vi "FFT Filt.vi"(0 "Filter in":refnum<class "Filter.lvclass">, 5 "Y":dbl[](array[numeric]), 9 "Fs (Hz)":dbl, 11 "error in (no error)":errorcluster) -> (4 "Filter out":refnum<class "Filter.lvclass">, 6 "Yfilt":dbl[](array[numeric]), 10 "Gain":dbl, 15 "error out":errorcluster)   [LabVIEW 2020, in "Filter.lvclass"]
uses:
  Filter.lvclass
  Filter.lvclass/Filter.ctl
  Utility VIs/Math VIs/FFT x(t) to dB,Degrees (1D).vi
  Utility VIs/Math VIs/Z to dB, degrees (1D).vi
  Utility VIs/Math VIs/Linear to dB (scalar).vi
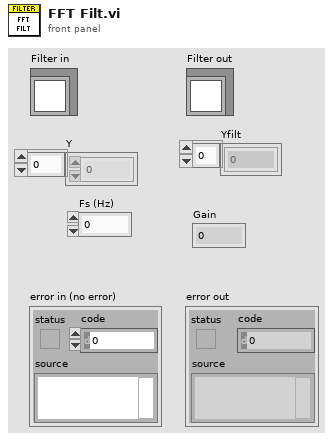
[diagram p1: front panel]
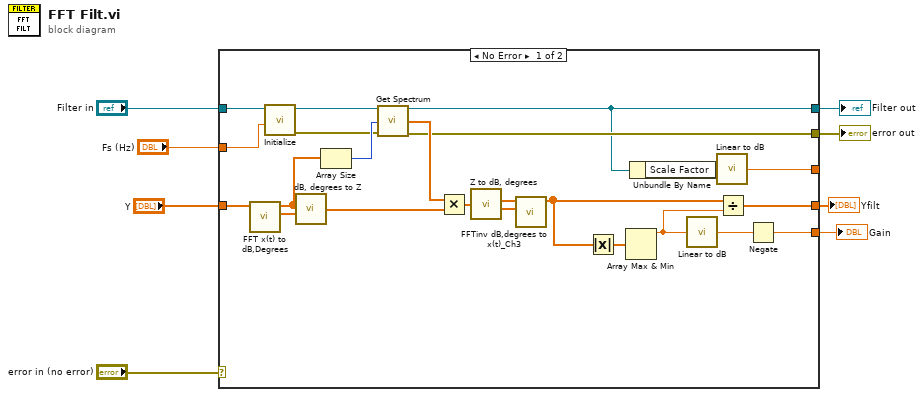
[diagram p0: block diagram]
diagram:
  n1 = case shown="No Error" "error in (no error)" {
    selector: "error in (no error)" -> [_ w33]
    tunnel: [w19 w33] -> w7
    tunnel: [w17 w32] -> w5
    tunnel: "Filter in" -> [w31 w32]
    tunnel: "Fs (Hz)" -> [w30 _]
    tunnel: "Y" -> [w28 _]
    tunnel: [w13 _] -> w2
    tunnel: [w12 _] -> _
    tunnel: [w9 _] -> w1
    frame No Error {
      n2 = call-poly "FFT x(t) to dB,Degrees.vi"("X"=w28) -> ("+Freq Phase of FFT (degrees)"=w26:dbl[], "+Freq. Mag of FFT (dB rms)"=w18:dbl[])  [unwired: 8 in, 1 out]
      n3 = call "Initialize.vi"("Fs (Hz)"=w30, "Filter in"=w31) -> ("error out"=w20:errorcluster, "Filter out"=w29:refnum<class "Filter.lvclass">)  [unwired: 8 in]
      n4 = call "dB, degrees to Z.vi"("Magnitude (dB)"=w18, "Phase (degrees)"=w26) -> ("Z"=w25:cdb[])  [unwired: 5 in]
      n5 = Array Size(array=w18) -> (size(s)=w27:i32)
      n6 = call "Get Spectrum.vi"("Filter in"=w29, "Npts"=w27, "error in (no error)"=w20) -> ("Filter out"=w17:refnum<class "Filter.lvclass">, "spectrum"=w24:cdb[], "error out"=w19:errorcluster)  [unwired: 10 in]
      n7 = Multiply(x=w24, y=w25) -> (x*y=w23:cdb[])
      n8 = call-poly "Z to dB, degrees.vi"("Z"=w23) -> ("Magnitude (dB)"=w22:dbl[], "Phase (degrees)"=w21:dbl[])  [unwired: 5 in]
      n9 = call "FFTinv dB,degrees to x(t)_Ch3.vi"("+Freq Phase of FFT (degrees)"=w21, "+Freq. Mag of FFT (rms dB)"=w22) -> ("X(t)"=w14:dbl[])  [unwired: 8 in, 1 out]
      n10 = Absolute Value(x=w14) -> (abs(x)=w15:dbl[])
      n11 = Array Max & Min(array=w15) -> (max value=w11:dbl)  [unwired: 3 out]
      n12 = Unbundle By Name(w17) -> ("Scale Factor"=w16:dbl)
      n13 = call-poly "Linear to dB.vi"("Linear"=w11) -> ("dB"=w10:dbl)
      n14 = call-poly "Linear to dB.vi"("Linear"=w16) -> ("dB"=w12:dbl)
      n15 = Divide(x=w14, y=w11) -> (x/y=w13:dbl[])
      n16 = Negate(x=w10) -> (-x=w9:dbl)
    }
    frame Error {
    }
  }
  "error out" <- w7
  "Filter out" <- w5
  "Yfilt" <- w2
  "Gain" <- w1
